vi "DFConfig Write Crawlitem Config.vi"(0 "Datafinder Indexer":T1={"repeat"=enum."daily", "enable_observer"=TRUE, "starttime"=timestamp(0 s since 1904-01-01), "timeout"=0}, 3 "Config In":string, 4 "Tag (\"\")":string) -> (5 "Config Out":string)   [LabVIEW 2011]
uses:
  DFConfig INDEXER.ctl
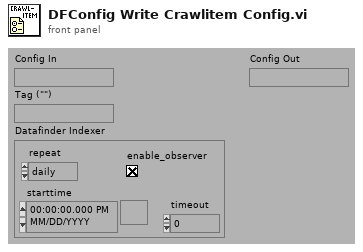
[diagram p1: front panel]
types:
  T1 = typedef "DFConfig INDEXER.ctl" = cluster{"repeat":enum16{"hourly", "daily", "weekly", "never"}, "enable_observer":bool, "starttime":timestamp, "timeout":i32}
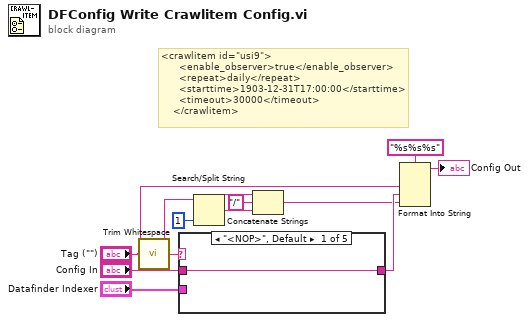
[diagram p0: block diagram]
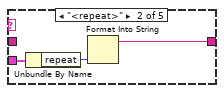
[diagram p2: hidden frame]
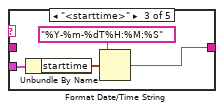
[diagram p3: hidden frame]
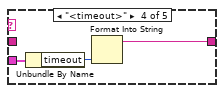
[diagram p4: hidden frame]
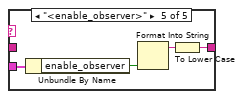
[diagram p5: hidden frame]
diagram:
  # "<crawlitem id=\"usi9\">\n      <enable_observer>true</enable_observer>\n      <repeat>daily</repeat>\n      <starttime>1903-12-31T17:00:00</starttime>\n      <timeout>30000</timeout>\n    </crawlitem>"
  n1 = call <vilib>:"Trim Whitespace.vi"("string"="Tag (\"\")") -> ("trimmed string"=w6:string)  [unwired: 1 in]
  n2 = case shown="\"<NOP>\", Default" w6 {
    tunnel: "Datafinder Indexer" -> [_ w15 w20 w23 w27]
    tunnel: [w13 w16 w19 w21 w24] -> w9
    tunnel: "Config In" -> [w13 _ _ _ _]
    frame "<NOP>", Default {
    }
    frame "<repeat>" {
      n3 = Unbundle By Name(w15) -> ("repeat"=w14:enum16{"hourly", "daily", "weekly", "never"})
      n4 = Format Into String(w14) -> (resulting string=w16:string)  [unwired: 3 in, 1 out]
    }
    frame "<starttime>" {
      n5 = Unbundle By Name(w20) -> ("starttime"=w18:timestamp)
      n6 = Format Date/Time String(time format string (%c)="%Y-%m-%dT%H:%M:%S", seconds (now)=w18) -> (date/time string=w19:string)  [unwired: 1 out]
    }
    frame "<timeout>" {
      n7 = Unbundle By Name(w23) -> ("timeout"=w22:i32)
      n8 = Format Into String(w22) -> (resulting string=w21:string)  [unwired: 3 in, 1 out]
    }
    frame "<enable_observer>" {
      n9 = Unbundle By Name(w27) -> ("enable_observer"=w26:bool)
      n10 = Format Into String(w26) -> (resulting string=w25:string)  [unwired: 3 in, 1 out]
      n11 = To Lower Case(string=w25) -> (all lower case string=w24:string)
    }
  }
  n12 = Search/Split String(string=w6, offset (0)=1) -> (substring before match=w5:string, match + rest of string=w4:string)  [unwired: 2 out]
  n13 = Concatenate Strings(w5, "/" ("string"), w4) -> (w3:string)
  n14 = Format Into String(format string="%s%s%s", "Tag (\"\")", w9, w3) -> (resulting string=→"Config Out":string)  [unwired: 2 in, 1 out]
